vi "U64 to I32 2D Array.vi"(2 "error in (no error)":errorcluster, 3 "U64":dbl[][](array[numeric])) -> (0 "error out":errorcluster, 1 "I32":i32[][](array[numeric]))   [LabVIEW 2017]
panel:
  # "LVHDF5 Toolkit\nCopyright (c) 2005-2013 by Jason D. Sommerville\nCopyright (c) 2014 by UPVI, LLC.\n\nThis use and distribution of this file is governed by the terms found in \nLICENSE.txt distributed with this toolkit and installed at\n <user.lib>\\_lvhdf5\\LICENSE.txt"
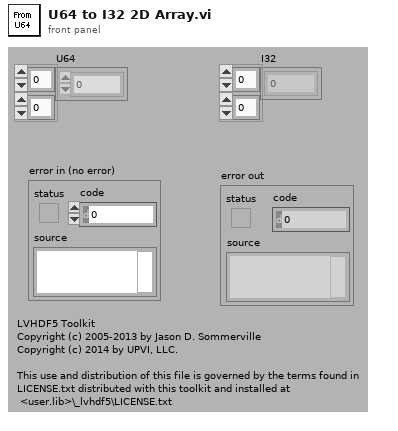
[diagram p1: front panel]
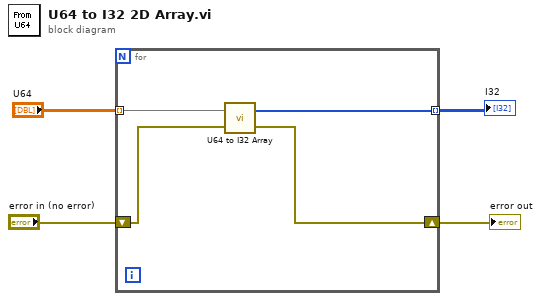
[diagram p0: block diagram]
diagram:
  n1 = for {
    tunnel: "U64" -> [w8] mode=indexing
    shift-right: [w6] -> w1
    shift-left: "error in (no error)" -> [w7]
    tunnel: [w5] -> w2 mode=indexing
    n2 = call <vilib>:"U64 to I32 Array.vi"("error in (no error)"=w7, "U64"=w8) -> ("error out"=w6:errorcluster, "I32"=w5:i32[])
  }
  "I32" <- w2
  "error out" <- w1
